vi "airport경로.vi"() -> ()   [LabVIEW 2014]
panel:
  out "경로":path
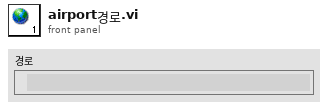
[diagram p1: front panel]
diagram:
